vi "Model.vi"(8 "error in":errorcluster, 10 "Queues":T2, 11 "Notifiers":T1) -> (0 "error out":errorcluster)   [LabVIEW 2014, in "Model.lvlib"]
uses:
  Model.lvlib
  support/Message Queue/Message Queue.lvlib
  TypeDefs/PL UI Refs.ctl
  TypeDefs/PL Settings.ctl
  TypeDefs/Model Data.ctl
  <vilib>/ErrorRing/Error Ring.xnode
  DAQ/DAQ.lvlib
  Support/Message Queue/Enqueue Message (Single).vi
  <vilib>/Utility/error.llb/Error Cluster From Error Code.vi
  Support/Global names.vi
  TypeDefs/UI/Line simulation.ctl
  Support/Message Queue/Message Cluster.ctl
  Support/Message Queue/All Message Queues.ctl
  Support/Notifiers/Notifiers.ctl
  Support/Notifiers/Notifiers.lvlib
panel:
  out "Barrel Number":i32
  out "BARREL FILLED":bool
  out "SPILL ALARM":bool
  out "OUTPUT":bool
  out "DOSING":bool
  out "INPUT":bool
  out "Flow [l/s]":dbl(knob) scale=0.0..30.0
  out "Fluid Level [l]":dbl(slide) scale=0.0..100.0
  out "Production line position":T3 max=100.0 scale=0.0..20.0
  out "Pump":bool
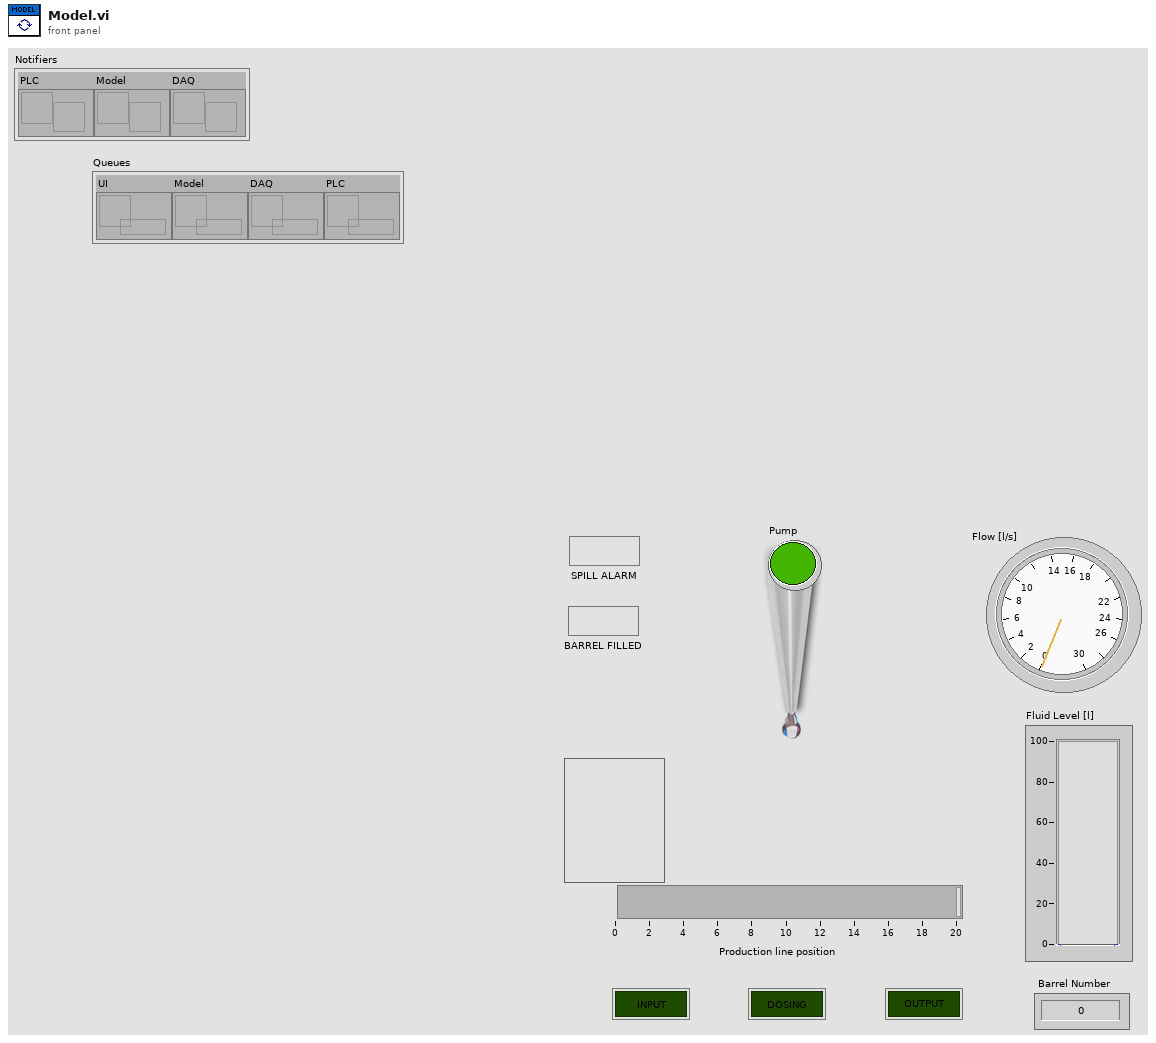
[diagram p1: front panel]
types:
  T1 = typedef "Notifiers.lvlib/Notifiers.ctl" = cluster{"PLC":refnum<notifier>, "Model":refnum<notifier>, "DAQ":refnum<notifier>}
  T2 = typedef "Message Queue.lvlib/All Message Queues.ctl" = cluster{"UI":refnum<queue>, "Model":refnum<queue>, "DAQ":refnum<queue>, "PLC":refnum<queue>}
  T3 = typedef "Model.lvlib/Line simulation.ctl" = dbl
  T4 = typedef "Model.lvlib/Model Data.ctl" = cluster{"Position":dbl, "Settings":T5, "Pump State":bool, "Fluid Flow":dbl, "Inpute Zone":bool, "Dosing Zone":bool, "Output Zone":bool, "UI Refs":T6, "Fluid Level":dbl, "Barrel Number":i32, "Spill Alarm":bool, "Level Alarm":bool, "millisecond timer value":u32, "Start simulation":bool}
  T5 = typedef "Model.lvlib/PL Settings.ctl" = cluster{"Length [m]":dbl, "Dose Zone Start":dbl, "Dose Zone  End":dbl, "Barrel Volume [l]":dbl, "Dosing level [l]":dbl}
  T6 = typedef "Model.lvlib/PL UI Refs.ctl" = cluster{"DOSING":refnum<vi>, "INPUT":refnum<vi>, "OUTPUT":refnum<vi>, "Pump":refnum<vi>, "Fluid Level [l]":refnum<vi>, "Flow [l/s]":refnum<vi>, "Production line":refnum<vi>, "SPILL":refnum<vi>, "LOW LEVEL":refnum<vi>, "Barrel Number":refnum<vi>}
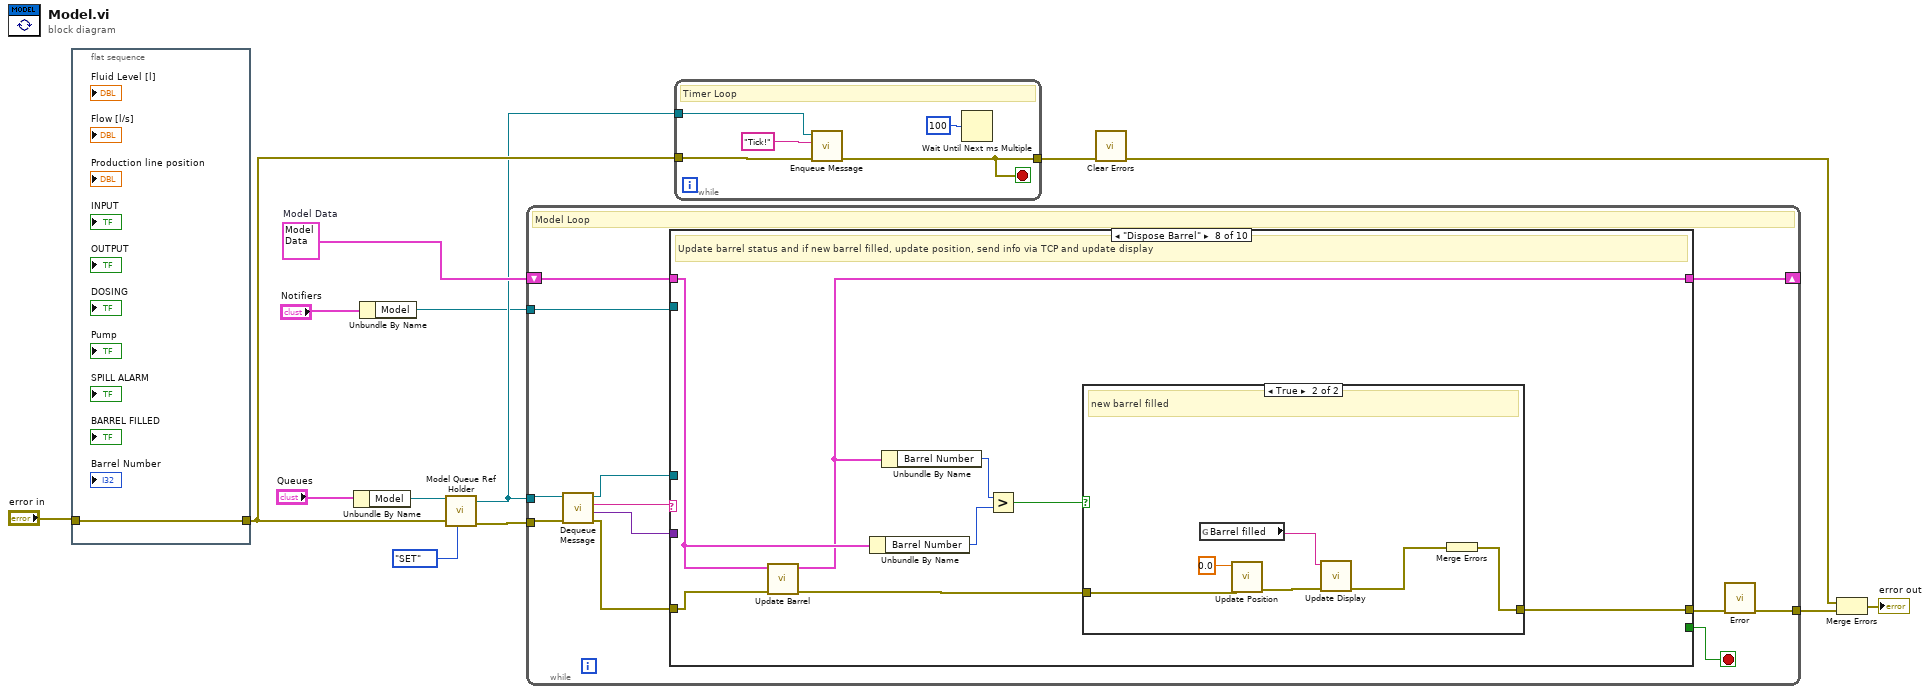
[diagram p0: block diagram]
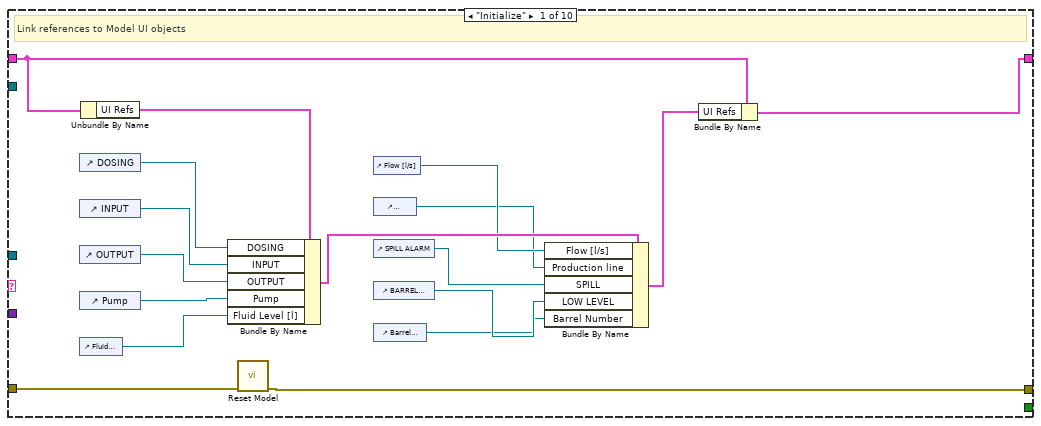
[diagram p2: hidden frame]
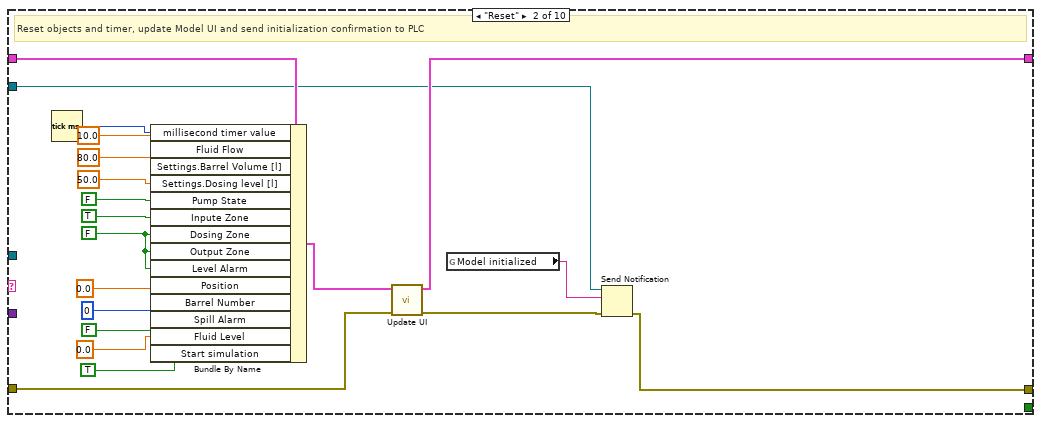
[diagram p3: hidden frame]
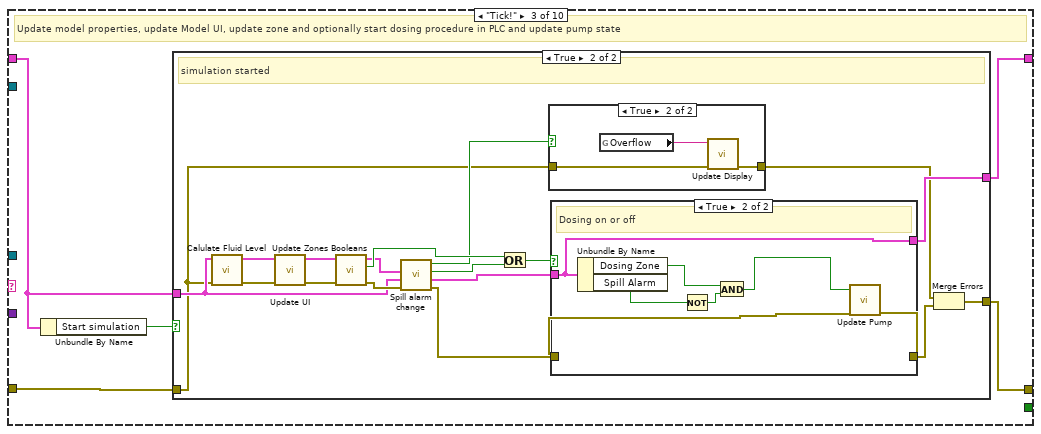
[diagram p4: hidden frame]
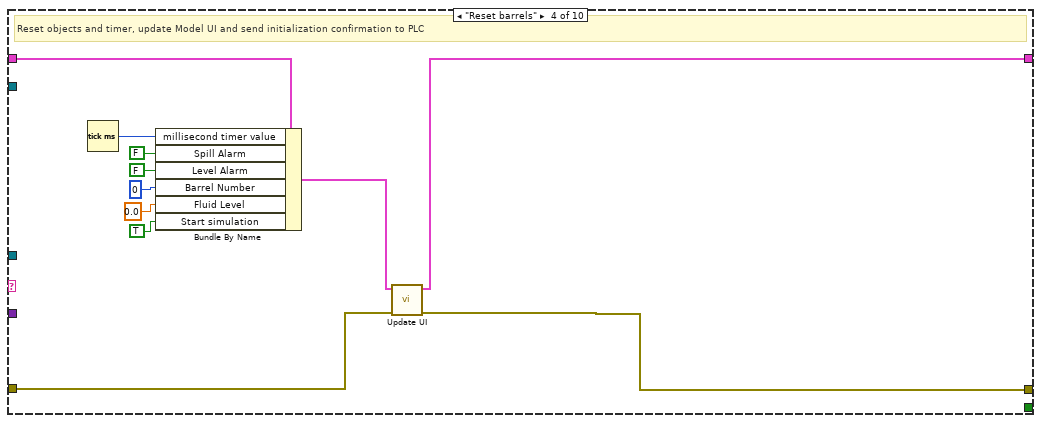
[diagram p8: hidden frame]
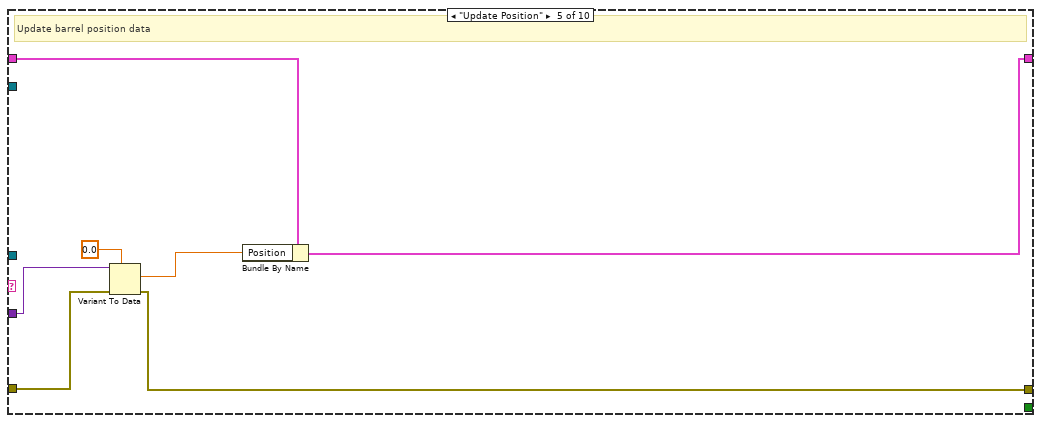
[diagram p9: hidden frame]
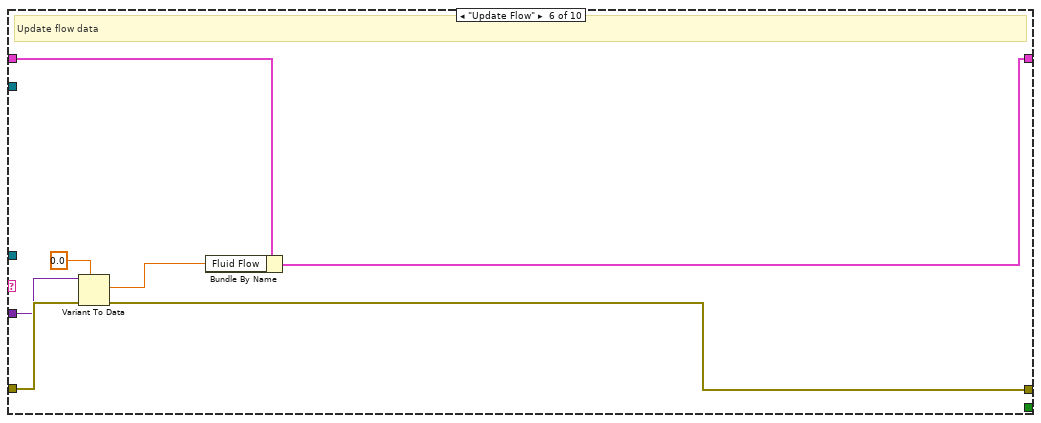
[diagram p10: hidden frame]
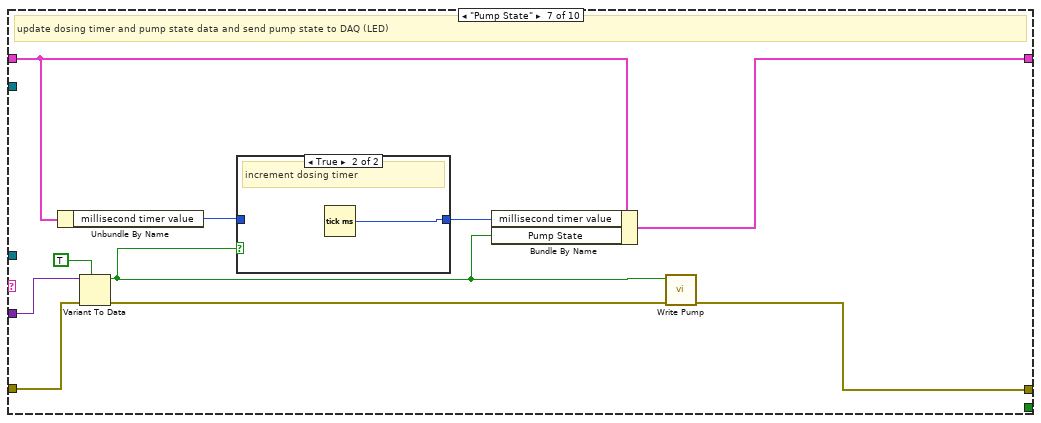
[diagram p11: hidden frame]
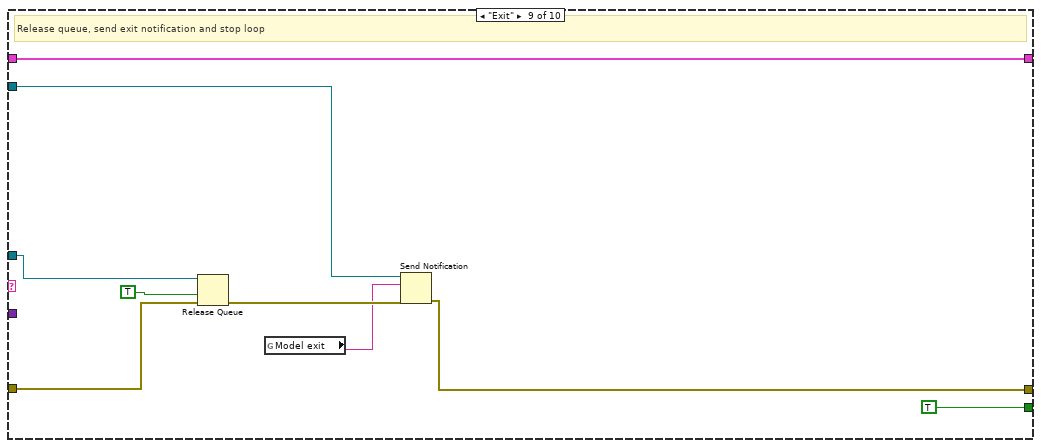
[diagram p14: hidden frame]
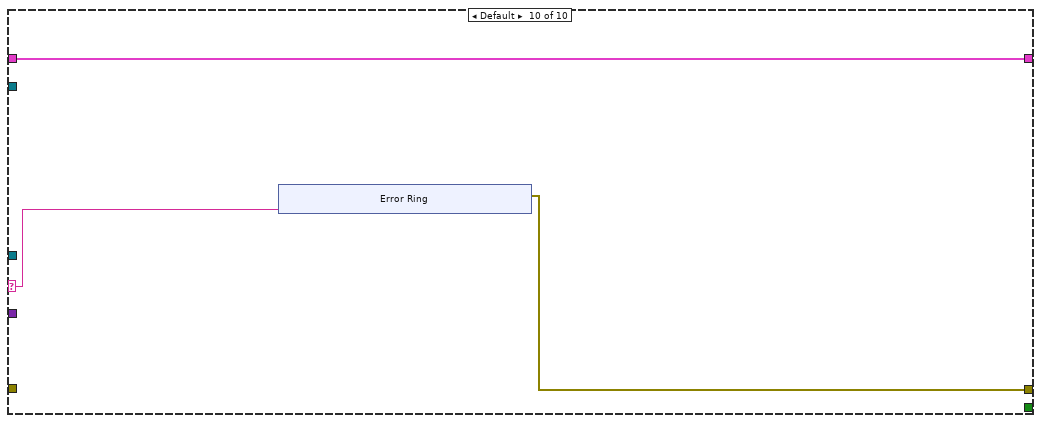
[diagram p15: hidden frame]
diagram:
  w12 = T4 {"Position"=0.0, "Settings"={"Length [m]"=20.0, "Dose Zone Start"=8.0, "Dose Zone  End"=12.0, "Barrel Volume [l]"=100.0, "Dosing level [l]"=90.0}, "Pump State"=FALSE, "Fluid Flow"=10.0, "Inpute Zone"=FALSE, "Dosing Zone"=FALSE, "Output Zone"=FALSE, "UI Refs"={"DOSING"=refnum, "INPUT"=refnum, "OUTPUT"=refnum, "Pump"=refnum, "Fluid Level [l]"=refnum, "Flow [l/s]"=refnum, "Production line"=refnum, "SPILL"=refnum, "LOW LEVEL"=refnum, "Barrel Number"=refnum}, "Fluid Level"=0.0, "Barrel Number"=0, "Spill Alarm"=FALSE, "Level Alarm"=FALSE, "millisecond timer value"=0, "Start simulation"=FALSE}  # Model Data
  n1 = flat-sequence {
    tunnel: "error in" -> [w15]
    tunnel: [w15] -> w11
    frame #0 {
    }
  }
  n2 = Unbundle By Name("Queues") -> ("Model"=w4:refnum<queue>)
  n3 = Unbundle By Name("Notifiers") -> ("Model"=w5:refnum<notifier>)
  n4 = call "Model Queue Ref Holder.vi"("Action"=enum16{"GET", "SET"}."SET", "error in"=w11, "Message Queue In"=w4) -> ("error out"=w10:errorcluster, "Input Message Queue"=w9:refnum<queue>)  [unwired: 7 in]
  n5 = while {
    tunnel: w9 -> [w27]
    shift-right: [w21] -> _
    shift-left: w12 -> [w22]
    tunnel: [w17] -> w1
    tunnel: w10 -> [w25]
    tunnel: w5 -> [w19]
    stop <- w20 stop-if-true
    # "Model Loop"
    n6 = call "Dequeue Message.vi"("error in (no error)"=w25, "Message Queue"=w27) -> ("error out"=w26:errorcluster, "Message Data"=w23:variant, "Message"=w24:string, "dup Message Queue"=w16:refnum<queue>)  [unwired: 6 in]
    n7 = case shown="\"Dispose Barrel\"" w24 {
      selector: w24 -> [_ _ _ _ _ _ _ _ _ w165]
      tunnel: w26 -> [w36 w55 w69 w111 w120 w127 w137 w147 w156 _]
      tunnel: [w35 w48 w68 w103 w114 w121 w133 w146 w157 w164] -> w18
      tunnel: w23 -> [_ _ _ _ w119 w126 w136 _ _ _]
      tunnel: w16 -> [_ _ _ _ _ _ _ _ w162 _]
      tunnel: w22 -> [w38 w64 w66 w113 w118 w125 w131 w145 w163 w166]
      tunnel: [w37 w54 w67 w110 w117 w124 w128 w144 w163 w166] -> w21
      tunnel: [_ _ _ _ _ _ _ _ TRUE ("Priority Message? (F)") _] -> w20
      tunnel: w19 -> [_ w47 _ _ _ _ _ _ w160 _]
      frame "Initialize" {
        # "Link references to Model UI objects"
        n8 = control-ref of="DOSING"() -> (w40:refnum<vi>)
        n9 = control-ref of="INPUT"() -> (w41:refnum<vi>)
        n10 = control-ref of="OUTPUT"() -> (w42:refnum<vi>)
        n11 = control-ref of="Pump"() -> (w43:refnum<vi>)
        n12 = control-ref of="Fluid Level [l]"() -> (w44:refnum<vi>)
        n13 = Unbundle By Name(w38) -> ("UI Refs"=w39:T6)
        n14 = Bundle By Name(cluster=w39, "DOSING"=w40, "INPUT"=w41, "OUTPUT"=w42, "Pump"=w43, "Fluid Level [l]"=w44) -> (w34:T6)
        n15 = call "Reset Model.vi"("error in"=w36) -> ("error out"=w35:errorcluster)  [unwired: 10 in]
        n16 = control-ref of="Flow [l/s]"() -> (w32:refnum<vi>)
        n17 = control-ref of="Production line"() -> (w31:refnum<vi>)
        n18 = control-ref of="SPILL ALARM"() -> (w30:refnum<vi>)
        n19 = control-ref of="BARREL FILLED"() -> (w29:refnum<vi>)
        n20 = control-ref of="Barrel Number"() -> (w28:refnum<vi>)
        n21 = Bundle By Name(cluster=w34, "Flow [l/s]"=w32, "Production line"=w31, "SPILL"=w30, "LOW LEVEL"=w29, "Barrel Number"=w28) -> (w33:T6)
        n22 = Bundle By Name(cluster=w38, "UI Refs"=w33) -> (w37:T4)
      }
      frame "Reset" {
        w58 = FALSE ("Inpute Zone")
        # "Reset objects and timer, update Model UI and send initialization confirmation to PLC"
        n23 = Tick Count (ms)() -> (millisecond timer value=w63:u32)
        n24 = Bundle By Name(cluster=w64, "millisecond timer value"=w63, "Fluid Flow"=10.0, "Settings.Barrel Volume [l]"=80.0, "Settings.Dosing level [l]"=50.0, "Pump State"=FALSE, "Inpute Zone"=TRUE, "Dosing Zone"=w58, "Output Zone"=w58, "Level Alarm"=w58, "Position"=0.0, "Barrel Number"=0, "Spill Alarm"=FALSE, "Fluid Level"=0.0, "Start simulation"=TRUE) -> (w56:T4)
        n25 = call "Update UI.vi"("error in (no error)"=w55, "Model Data in"=w56) -> ("error out"=w46:errorcluster, "Model Data out"=w54:T4)  [unwired: 8 in]
        n26 = global read "Global names.vi" "Model initialized"() -> (w45:string)
        n27 = Send Notification(notification=w45, notifier=w47, error in (no error)=w46) -> (error out=w48:errorcluster)  [unwired: 1 out]
      }
      frame "Tick!" {
        # "Update model properties, update Model UI, update zone and optionally start dosing procedure in PLC and update pump state"
        n28 = Unbundle By Name(w66) -> ("Start simulation"=w65:bool)
        n29 = case shown="True" w65 {
          tunnel: w69 -> [w71 w73]
          tunnel: w66 -> [w70 w74]
          tunnel: [w71 w84] -> w68
          tunnel: [w70 w78] -> w67
          frame False {
            # "simulation model not initialized yet"
          }
          frame True {
            # "simulation started"
            n30 = call "Calulate Fluid Level.vi"("error in (no error)"=w73, "Model Data"=w74) -> ("error out"=w89:errorcluster, "Model Data Out"=w86:T4)  [unwired: 8 in]
            n31 = call "Update UI.vi"("error in (no error)"=w89, "Model Data in"=w86) -> ("error out"=w88:errorcluster, "Model Data out"=w87:T4)  [unwired: 8 in]
            n32 = call "Update Zones Booleans.vi"("error in (no error)"=w88, "Model Data in"=w87) -> ("error out"=w82:errorcluster, "Zone change?"=w80:bool, "Model Data out"=w77:T4)  [unwired: 7 in]
            n33 = call "Spill alarm change.vi"("error in"=w82, "Model Data before update"=w74, "Model Data after update"=w77) -> ("error out"=w81:errorcluster, "Model Data after update out"=w76:T4, "Spill alarm value change"=w79:bool, "Spill alarm turned on"=w75:bool)  [unwired: 5 in]
            n34 = Or(x=w80, y=w79) -> (x .or. y?=w83:bool)
            n35 = case shown="True" w75 {
              tunnel: w73 -> [w90 w93]
              tunnel: [w90 w92] -> w72
              frame False {
              }
              frame True {
                n36 = global read "Global names.vi" "Overflow"() -> (w91:string)
                n37 = call "Update Display.vi"("error in"=w93, "Message string"=w91) -> ("error out"=w92:errorcluster)  [unwired: 9 in]
              }
            }
            n38 = case shown="True" w83 {
              tunnel: w76 -> [w94 w97]
              tunnel: w81 -> [w95 w96]
              tunnel: [w95 w99] -> w85
              tunnel: [w94 w97] -> w78
              frame False {
                # "No dosing change"
              }
              frame True {
                # "Dosing on or off"
                n39 = Unbundle By Name(w97) -> ("Dosing Zone"=w100:bool, "Spill Alarm"=w102:bool)
                n40 = Not(x=w102) -> (.not. x?=w101:bool)
                n41 = And(x=w100, y=w101) -> (x .and. y?=w98:bool)
                n42 = call "Update Pump.vi"("error in (no error)"=w96, "Pump State"=w98) -> ("error out"=w99:errorcluster)  [unwired: 9 in]
              }
            }
            n43 = Merge Errors(w72, w85) -> (w84:errorcluster)
          }
        }
      }
      frame "Reset barrels" {
        # "Reset objects and timer, update Model UI and send initialization confirmation to PLC"
        n44 = Tick Count (ms)() -> (millisecond timer value=w104:u32)
        n45 = Bundle By Name(cluster=w113, "millisecond timer value"=w104, "Spill Alarm"=FALSE, "Level Alarm"=FALSE, "Barrel Number"=0, "Fluid Level"=0.0, "Start simulation"=TRUE) -> (w112:T4)
        n46 = call "Update UI.vi"("error in (no error)"=w111, "Model Data in"=w112) -> ("error out"=w103:errorcluster, "Model Data out"=w110:T4)  [unwired: 8 in]
      }
      frame "Update Position" {
        # "Update barrel position data"
        n47 = Variant To Data(error in=w120, type=0.0, Variant=w119) -> (data=w116:dbl, error out=w114:errorcluster)
        n48 = Bundle By Name(cluster=w118, "Position"=w116) -> (w117:T4)
      }
      frame "Update Flow" {
        # "Update flow data"
        n49 = Variant To Data(error in=w127, type=0.0, Variant=w126) -> (data=w122:dbl, error out=w121:errorcluster)
        n50 = Bundle By Name(cluster=w125, "Fluid Flow"=w122) -> (w124:T4)
      }
      frame "Pump State" {
        # "update dosing timer and pump state data and send pump state to DAQ (LED)"
        n51 = Unbundle By Name(w131) -> ("millisecond timer value"=w132:u32)
        n52 = Variant To Data(error in=w137, type=TRUE, Variant=w136) -> (data=w129:bool, error out=w134:errorcluster)
        n53 = case shown="True" w129 {
          tunnel: w132 -> [w138 _]
          tunnel: [w138 w139] -> w130
          frame False {
            # "pause dosing timer"
          }
          frame True {
            # "increment dosing timer"
            n54 = Tick Count (ms)() -> (millisecond timer value=w139:u32)
          }
        }
        n55 = Bundle By Name(cluster=w131, "millisecond timer value"=w130, "Pump State"=w129) -> (w128:T4)
        n56 = call "Write Pump.vi"("error in"=w134, "Pump state"=w129) -> ("error out"=w133:errorcluster)  [unwired: 9 in]
      }
      frame "Dispose Barrel" {
        # "Update barrel status and if new barrel filled, update position, send info via TCP and update display"
        n57 = call "Update Barrel.vi"("error in (no error)"=w147, "PL Model Data in"=w145) -> ("error out"=w140:errorcluster, "PL Model Data out"=w144:T4)  [unwired: 8 in]
        n58 = Unbundle By Name(w145) -> ("Barrel Number"=w143:i32)
        n59 = Unbundle By Name(w144) -> ("Barrel Number"=w141:i32)
        n60 = Greater?(x=w141, y=w143) -> (0:w142:bool)
        n61 = case shown="True" w142 {
          tunnel: w140 -> [w148 w152]
          tunnel: [w148 w150] -> w146
          frame False {
          }
          frame True {
            # "new barrel filled"
            n62 = global read "Global names.vi" "Barrel filled"() -> (w149:string)
            n63 = call "Update Position.vi"("error in"=w152, "Position"=0.0) -> ("error out"=w154:errorcluster)  [unwired: 9 in]
            n64 = call "Update Display.vi"("error in"=w154, "Message string"=w149) -> ("error out"=w151:errorcluster)  [unwired: 9 in]
            n65 = Merge Errors(w151) -> (w150:errorcluster)
          }
        }
      }
      frame "Exit" {
        # "Release queue, send exit notification and stop loop"
        n66 = Release Queue(queue=w162, force destroy? (F)=TRUE, error in (no error)=w156) -> (error out=w161:errorcluster)  [unwired: 2 out]
        n67 = global read "Global names.vi" "Model exit"() -> (w155:string)
        n68 = Send Notification(notification=w155, notifier=w160, error in (no error)=w161) -> (error out=w157:errorcluster)  [unwired: 1 out]
      }
      frame Default {
        n69 = xnode "Error Ring"("parameter 0"=w165) -> ("error out"=w164:errorcluster)
      }
    }
    n70 = call "Error.vi"("error in"=w18) -> ("error out"=w17:errorcluster)  [unwired: 10 in]
  }
  n71 = while {
    tunnel: w9 -> [w177]
    tunnel: [w174] -> w8
    tunnel: w11 -> [w175]
    stop <- w174 stop-if-true
    # "Timer Loop"
    n72 = call-poly "Enqueue Message.vi"("error in (no error)"=w175, "Message"="Tick!", "Message Queue"=w177) -> ("error out"=w174:errorcluster)  [unwired: 7 in, 1 out]
    n73 = Wait Until Next ms Multiple(millisecond multiple=u32 100) -> ()  [unwired: 1 out]
  }
  n74 = call <vilib>:"Clear Errors.vi"("error in (no error)"=w8) -> ("error out"=w7:errorcluster)  [unwired: 5 in, 1 out]
  n75 = Merge Errors(w7, w1) -> (→"error out":errorcluster)
